vi "Convert Package Attribute Cluster to 2D String.vi"(8 "error in (no error)":errorcluster, 10 "package attributes (cluster)":T1) -> (0 "error out":errorcluster, 2 "package attributes (2D string)":string[][](table))   [LabVIEW 2014, in "NIPM_API.lvlib"]
doc: "Converts the package attribute cluster data type into a 2D string array. The default output is Table (2D string) indicator.\n\nUse this VI when you need to visualize package attribute values better in a Table indicator instead of a cluster indicator."
uses:
  NIPM_API.lvlib
  _support/package attributes.ctl
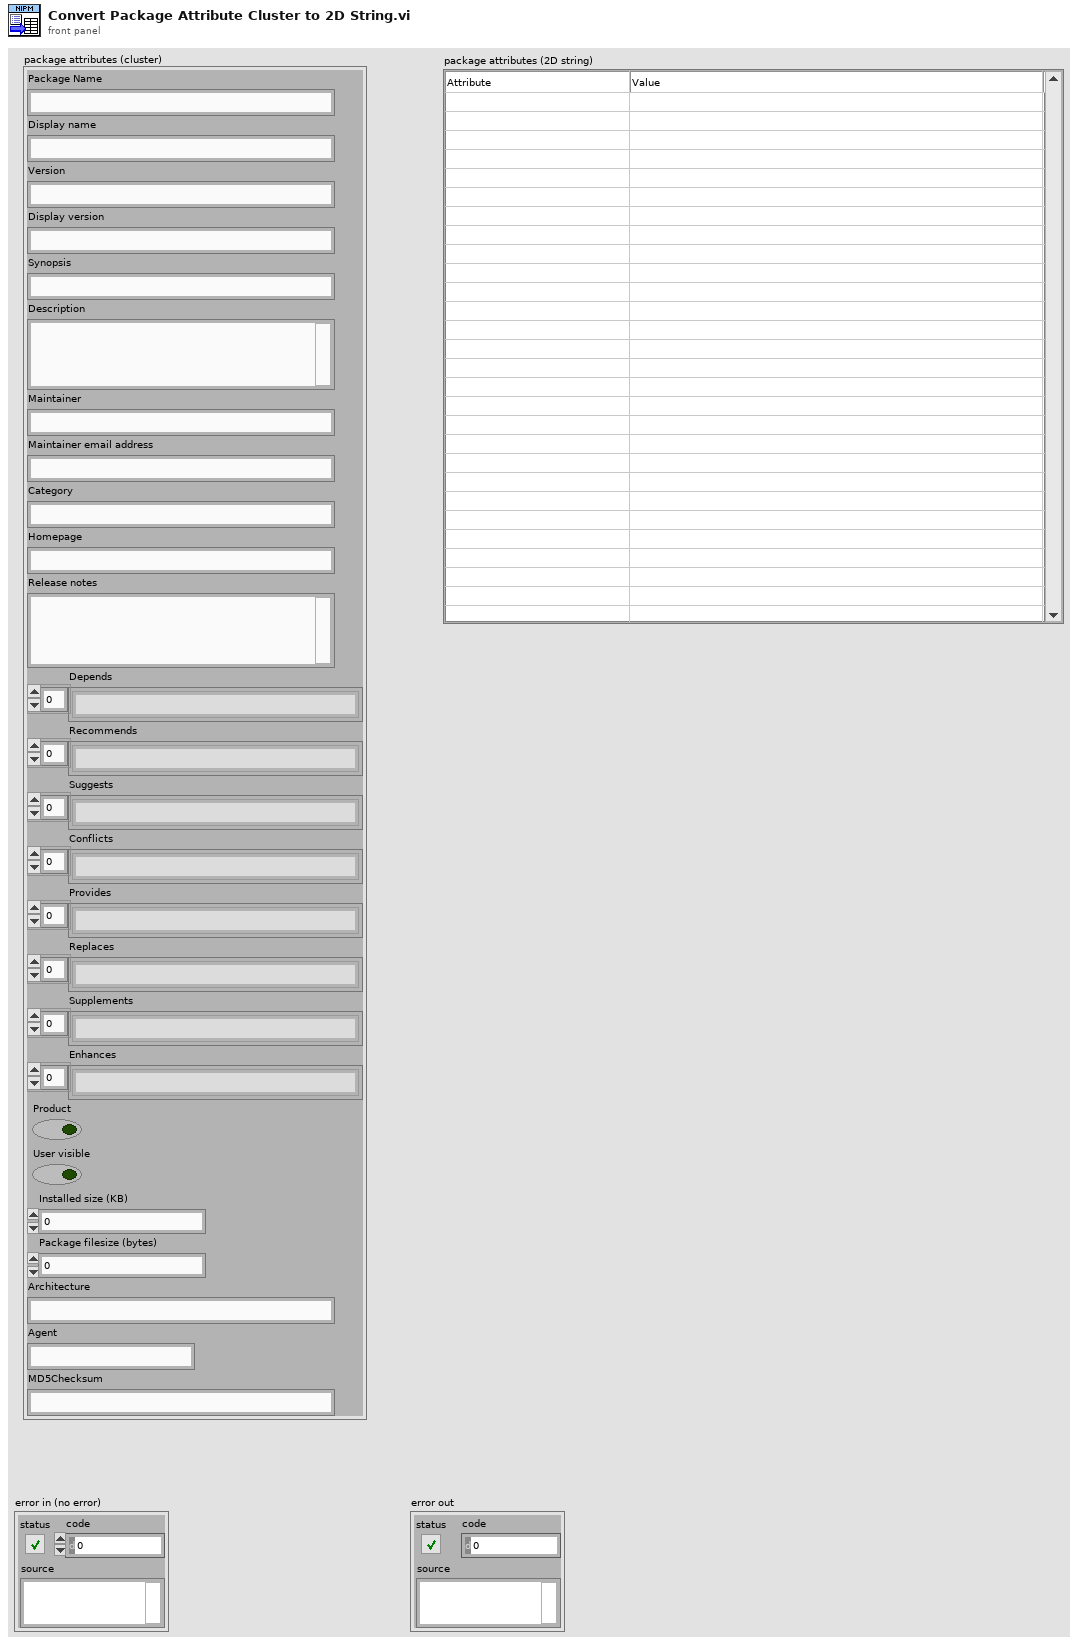
[diagram p1: front panel]
types:
  T1 = typedef "NIPM_API.lvlib/package attributes.ctl" = cluster{"Package Name":string, "Display name":string, "Version":string, "Display version":string, "Synopsis":string, "Description":string, "Maintainer":string, "Maintainer email address":string, "Category":string, "Homepage":string, "Release notes":string, "Depends":string[], "Recommends":string[], "Suggests":string[], "Conflicts":string[], "Provides":string[], "Replaces":string[], "Supplements":string[], "Enhances":string[], "Product":bool, "User visible":bool, "Installed size (KB)":u64, "Package filesize (bytes)":u64, "Architecture":string, "Agent":string, "MD5Checksum":string}
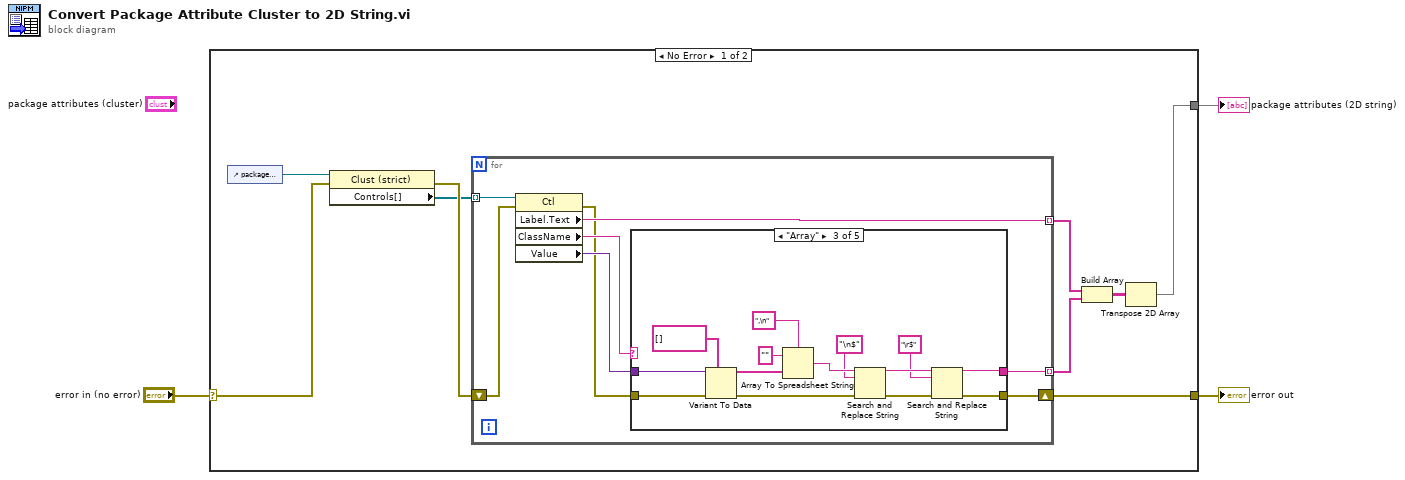
[diagram p0: block diagram]
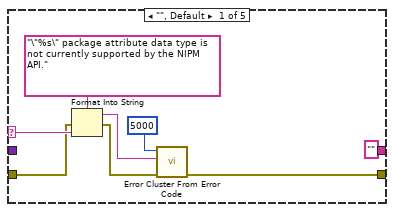
[diagram p2: hidden frame]
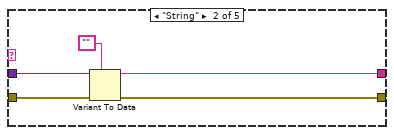
[diagram p3: hidden frame]
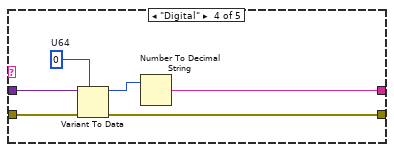
[diagram p4: hidden frame]
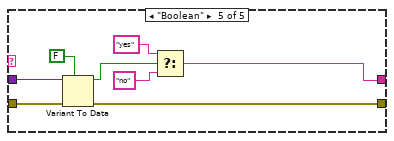
[diagram p5: hidden frame]
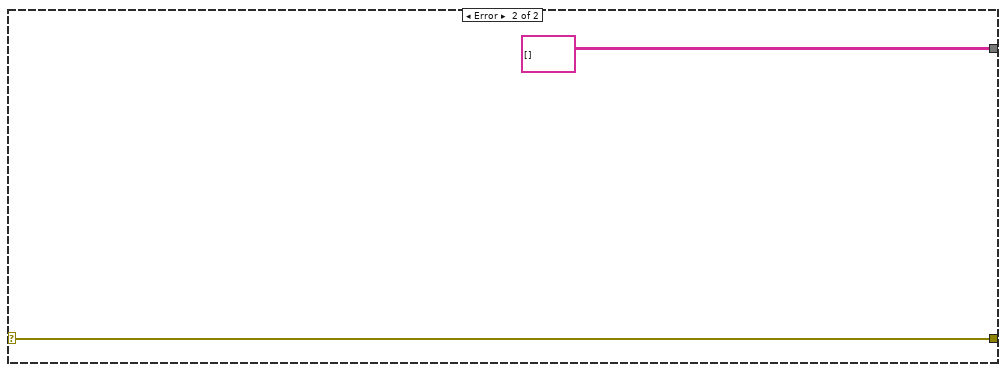
[diagram p6: hidden frame]
diagram:
  n1 = case shown="No Error" "error in (no error)" {
    selector: "error in (no error)" -> [w12 w63]
    tunnel: [w11 w63] -> w2
    tunnel: [w4 string[][] []] -> w1
    frame No Error {
      n2 = control-ref of="package attributes (cluster)"() -> (w5:refnum<vi>)
      n3 = property class="Clust (strict)"(reference=w5, error in=w12) -> (error out=w10:errorcluster, "Controls[]"=w9:refnum<vi>[])  [unwired: 1 out]
      n4 = for {
        tunnel: w9 -> [w20] mode=indexing
        tunnel: [w19] -> w8 mode=indexing
        tunnel: [w16] -> w7 mode=indexing
        shift-right: [w13] -> w11
        shift-left: w10 -> [w15]
        n5 = property class="Ctl"(reference=w20, error in=w15) -> (error out=w14:errorcluster, "Label.Text"=w19:string, "ClassName"=w18:string, "Value"=w17:variant)  [unwired: 1 out]
        n6 = case shown="\"Array\"" w18 {
          selector: w18 -> [w25 _ _ _ _]
          tunnel: w17 -> [_ w33 w46 w53 w61]
          tunnel: ["" ("spreadsheet string") w31 w35 w50 w56] -> w16
          tunnel: w14 -> [w22 w30 w45 w49 w55]
          tunnel: [w27 w29 w34 w48 w54] -> w13
          frame "", Default {
            n7 = Format Into String(format string="\"%s\" package attribute data type is not currently supported by the NIPM API.", error in=w22, w25) -> (resulting string=w23:string, error out=w21:errorcluster)  [unwired: 1 in]
            n8 = call <vilib>:"Error Cluster From Error Code.vi"("error in (no error)"=w21, "error message (\"\")"=w23, "error code (0)"=5000) -> ("error out"=w27:errorcluster)  [unwired: 6 in]
          }
          frame "String" {
            n9 = Variant To Data(error in=w30, type="", Variant=w33) -> (data=w31:string, error out=w29:errorcluster)
          }
          frame "Array" {
            n10 = Variant To Data(error in=w45, type=string[] [], Variant=w46) -> (data=w36:string[], error out=w37:errorcluster)
            n11 = Array To Spreadsheet String(delimiter (Tab)=",\n", array=w36, 3:"" ("format string")) -> (spreadsheet string=w42:string)
            n12 = Search and Replace String(input string=w42, search string="\n$", error in=w37) -> (result string=w39:string, error out=w40:errorcluster)  [unwired: 5 in, 2 out]
            n13 = Search and Replace String(input string=w39, search string="\r$", error in=w40) -> (result string=w35:string, error out=w34:errorcluster)  [unwired: 5 in, 2 out]
          }
          frame "Digital" {
            w52 = u64 0  # U64
            n14 = Variant To Data(error in=w49, type=w52, Variant=w53) -> (data=w51:u64, error out=w48:errorcluster)
            n15 = Number To Decimal String(number=w51) -> (decimal integer string=w50:string)  [unwired: 1 in]
          }
          frame "Boolean" {
            n16 = Variant To Data(error in=w55, type=FALSE, Variant=w61) -> (data=w59:bool, error out=w54:errorcluster)
            n17 = Select(t="yes", s=w59, f="no") -> (s? t:f=w56:string)
          }
        }
      }
      n18 = Build Array(w8, w7) -> (w6:string[][])
      n19 = Transpose 2D Array(2D array=w6) -> (transposed array=w4:string[][])
    }
    frame Error {
    }
  }
  "error out" <- w2
  "package attributes (2D string)" <- w1
